vi "AggregateReports.vi"(6 "Additional In":T1 {"Synx" format="%#_4g"}, 11 "Aggregated In":T1 {"Synx" format="%#_4g"}) -> (3 "Aggregated Out":T1 {"Synx" format="%#_4g"})   [LabVIEW 2017, in "AppPlugins.lvlib" / "AppPluginsBase.lvclass"]
uses:
  AppPluginsBase.lvclass
  EventPlugins/EventPluginBaseClass/TypeDefs/clEvtReportArray.ctl
  EventPlugins/EventPluginBaseClass/TypeDefs/clEvtReport.ctl
  EventPlugins/EventPluginBaseClass/EventPluginBaseClass.lvclass
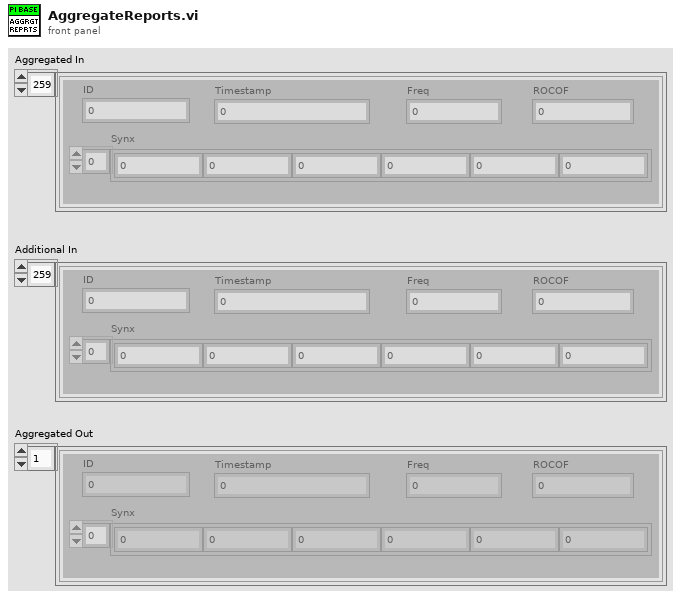
[diagram p1: front panel]
types:
  T1 = typedef "EventPlugins.lvlib/EventPluginBaseClass.lvclass/clEvtReportArray.ctl" = T2[]
  T2 = typedef "EventPlugins.lvlib/EventPluginBaseClass.lvclass/clEvtReport.ctl" = cluster{"Timestamp":dbl, "Synx":cdb[], "Freq":dbl, "ROCOF":dbl, "ID":i16}
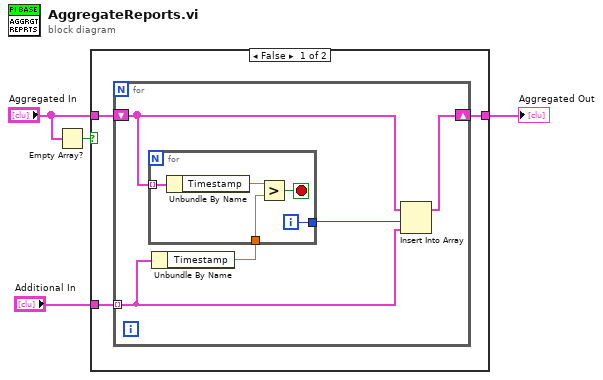
[diagram p0: block diagram]
diagram:
  n1 = Empty Array?(array="Aggregated In") -> (empty?=w1:bool)
  n2 = case shown="False" w1 {
    tunnel: "Additional In" -> [w7 w18]
    tunnel: [w6 w18] -> w3
    tunnel: "Aggregated In" -> [w5 _]
    frame False {
      n3 = for {
        tunnel: w7 -> [w10] mode=indexing
        shift-right: [w9] -> w6
        shift-left: w5 -> [w8]
        n4 = Unbundle By Name(w10) -> ("Timestamp"=w12:dbl)
        n5 = for {
          tunnel: w8 -> [w17] mode=indexing
          tunnel: w12 -> [w15]
          tunnel: [w13] -> w11
          i -> [w13]
          stop <- w14 stop-if-true
          n6 = Unbundle By Name(w17) -> ("Timestamp"=w16:dbl)
          n7 = Greater?(x=w16, y=w15) -> (0:w14:bool)
        }
        n8 = Insert Into Array(array=w8, index=w11, new element=w10) -> (w9:T1)
      }
    }
    frame True {
    }
  }
  "Aggregated Out" <- w3
